vi "Modify Object Owner.vi"(6 "timeout (100 ms)":i32, 10 "UniqueName Object":refnum<class "UniqueName.lvclass">, 11 "New Parent Fully Qualified Name":string) -> (0 "timed out":bool, 1 "operation complete":bool, 2 "Modified UniqueName Object":refnum<class "UniqueName.lvclass">)   [LabVIEW 2014, in "UniqueName.lvlib" / "UniqueName.lvclass"]
uses:
  UniqueName.lvclass
  Command.ctl
  UniquenessCriteria/UniquenessCriteria.lvclass/UniquenessCriteria.ctl
  UniqueName.lvclass/UniqueName.ctl
  Key.ctl
  UniquenessCriteria/UniquenessCriteria.lvclass
  NameIncrementAlgorithm/StringIncrementAlgorithm.lvclass
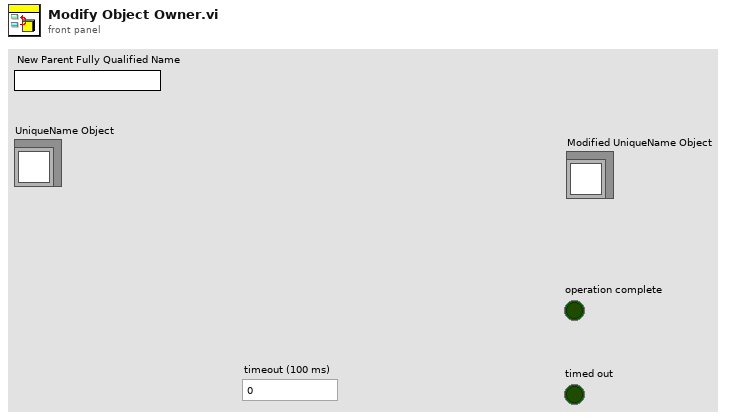
[diagram p1: front panel]
types:
  T1 = typedef "UniqueName.lvlib/UniqueName.lvclass/Command.ctl" = enum16{"Get", "Get All", "Set", "Delete", "Get Status", "Init", "Reserve Ownership", "Release Ownership", "Lock", "Unlock"}
  T2 = typedef "UniqueName.lvlib/UniqueName.lvclass/RegistryStatus.ctl" = cluster{"Registry Configuration":T3, "Registry Owned":bool, "Write-Protected":bool, "Owned":bool, "Released":bool, "Locked":bool, "Unlocked":bool}
  T3 = typedef "UniqueName.lvlib/UniqueName.lvclass/RegistryConfiguration.ctl" = cluster{"Delimiter":refnum<class "Delimiter.lvclass">, "RandomStringGenerator":refnum<class "RandomStringGenerator.lvclass">, "UniquenessCriteria":refnum<class "UniquenessCriteria.lvclass">, "StringIncrement":refnum<class "StringIncrementAlgorithm.lvclass">}
  T4 = typedef "UniqueName.lvlib/UniqueName.lvclass/Key.ctl" = enum16{"Fully Qualified Name", "Unique Name", "Given Name", "Parent Fully Qualified Name"}
  T5 = typedef "UniqueName.lvlib/UniquenessCriteria.lvclass/Criteria.ctl" = enum16{"Globally-Unique Fully Qualified Name", "Globally-Unique Name"}
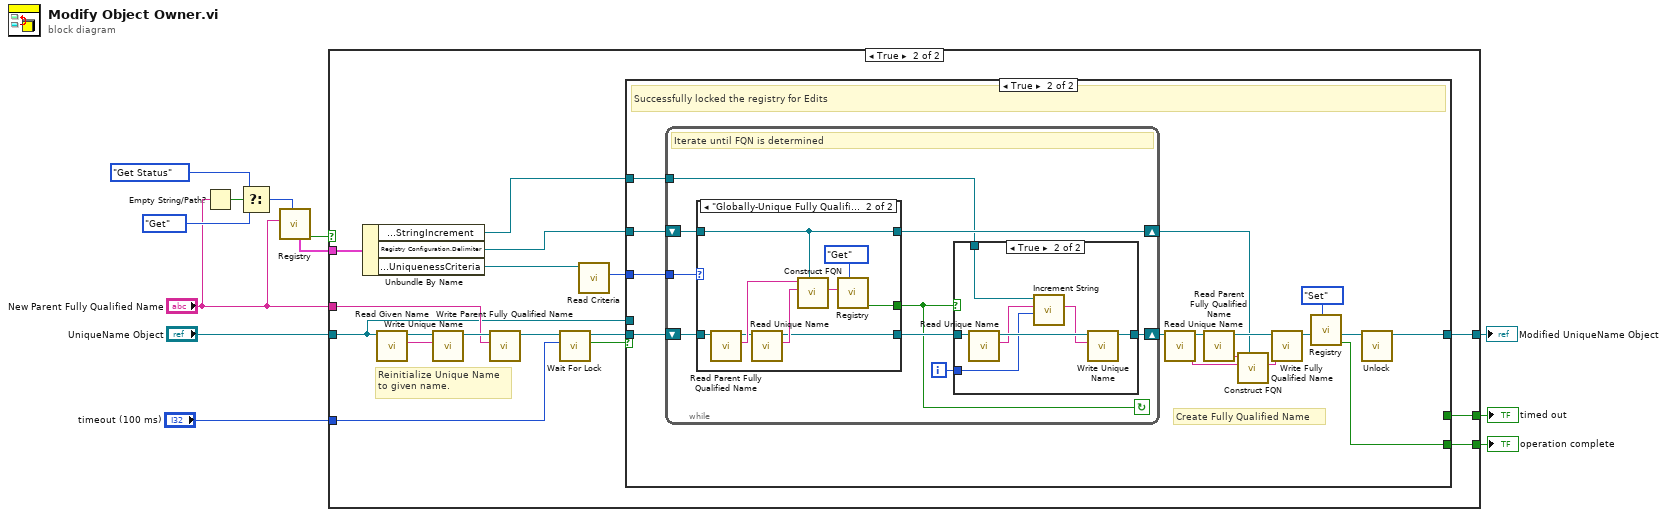
[diagram p0: block diagram]
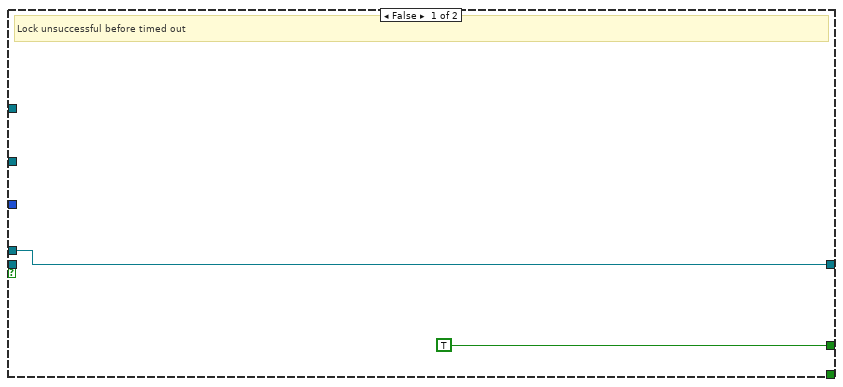
[diagram p3: hidden frame]
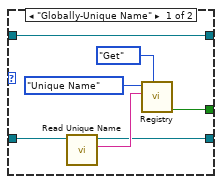
[diagram p5: hidden frame]
diagram:
  n1 = Empty String/Path?(string/path="New Parent Fully Qualified Name") -> (empty?=w8:bool)
  n2 = Select(t=Command."Get Status" ("Command (Get)"), s=w8, f=Command."Get" ("Command (Get)")) -> (s? t:f=w5:T1)
  n3 = call "Registry.vi"("Command (Get)"=w5, "Search term (Get & Delete Operations)"="New Parent Fully Qualified Name") -> ("Found or Completed?"=w3:bool, "Registry Status"=w10:T2)  [unwired: 5 in, 3 out]
  n4 = case shown="True" w3 {
    tunnel: [w13 w29] -> w12
    tunnel: [_ w27] -> w11
    tunnel: w10 -> [_ w26]
    tunnel: "timeout (100 ms)" -> [_ w24]
    tunnel: "UniqueName Object" -> [w13 w14]
    tunnel: "New Parent Fully Qualified Name" -> [_ w18]
    tunnel: [_ w17] -> w2
    frame False {
    }
    frame True {
      # "Reinitialize Unique Name\nto given name."
      n5 = Unbundle By Name(w26) -> ("Registry Configuration.StringIncrement"=w21:refnum<class "StringIncrementAlgorithm.lvclass">, "Registry Configuration.Delimiter"=w22:refnum<class "Delimiter.lvclass">, "Registry Configuration.UniquenessCriteria"=w23:refnum<class "UniquenessCriteria.lvclass">)
      n6 = call "Read Given Name.vi"("UniqueName in"=w14) -> ("Given Name"=w15:string, "UniqueName out"=w16:refnum<class "UniqueName.lvclass">)  [unwired: 9 in]
      n7 = call "Write Unique Name.vi"("Unique Name"=w15, "UniqueName in"=w16) -> ("UniqueName out"=w30:refnum<class "UniqueName.lvclass">)  [unwired: 9 in]
      n8 = call "Write Parent Fully Qualified Name.vi"("Parent Fully Qualified Name"=w18, "UniqueName in"=w30) -> ("UniqueName out"=w19:refnum<class "UniqueName.lvclass">)  [unwired: 9 in]
      n9 = call "Wait For Lock.vi"("timeout (100 ms)"=w24, "UniqueName in"=w19) -> ("Locked"=w28:bool, "UniqueName out"=w20:refnum<class "UniqueName.lvclass">)  [unwired: 8 in]
      n10 = call "Read Criteria.vi"("UniquenessCriteria in"=w23) -> ("Criteria"=w25:T5)  [unwired: 9 in, 1 out]
      n11 = case shown="True" w28 {
        tunnel: w25 -> [_ w47]
        tunnel: w20 -> [_ w40]
        tunnel: [w31 w37] -> w29
        tunnel: [TRUE _] -> w27
        tunnel: w22 -> [_ w36]
        tunnel: w21 -> [_ w35]
        tunnel: [_ w33] -> w17
        tunnel: w14 -> [w31 _]
        frame False {
          # "Lock unsuccessful before timed out"
        }
        frame True {
          # "Create Fully Qualified Name"
          # "Successfully locked the registry for Edits"
          n12 = while {
            tunnel: w47 -> [w57]
            shift-right: [w55] -> w43
            shift-left: w40 -> [w54]
            shift-right: [w51] -> w39
            shift-left: w36 -> [w52]
            tunnel: w35 -> [w50]
            i -> [w49]
            stop <- w53 continue-if-true
            # "Iterate until FQN is determined"
            n13 = case shown="\"Globally-Unique Fully Qualified Name\"" w57 {
              tunnel: [w70 w80] -> w53
              tunnel: w54 -> [w69 w75]
              tunnel: [w67 w73] -> w56
              tunnel: w52 -> [w66 w76]
              tunnel: [w66 w76] -> w51
              frame "Globally-Unique Name" {
                n14 = call "Read Unique Name.vi"("UniqueName in"=w69) -> ("Unique Name"=w68:string, "UniqueName out"=w67:refnum<class "UniqueName.lvclass">)  [unwired: 9 in]
                n15 = call "Registry.vi"("Command (Get)"=Command."Get", "Search term (Get & Delete Operations)"=w68, "Key (FQN)"=Key."Unique Name") -> ("Found or Completed?"=w70:bool)  [unwired: 4 in, 4 out]
              }
              frame "Globally-Unique Fully Qualified Name" {
                n16 = call "Read Parent Fully Qualified Name.vi"("UniqueName in"=w75) -> ("Parent Fully Qualified Name"=w78:string, "UniqueName out"=w74:refnum<class "UniqueName.lvclass">)  [unwired: 9 in]
                n17 = call "Read Unique Name.vi"("UniqueName in"=w74) -> ("Unique Name"=w77:string, "UniqueName out"=w73:refnum<class "UniqueName.lvclass">)  [unwired: 9 in]
                n18 = call "Construct FQN.vi"("Delimiter"=w76, "Name"=w77, "Parent FQN"=w78) -> ("FQN"=w79:string)  [unwired: 8 in]
                n19 = call "Registry.vi"("Command (Get)"=Command."Get", "Search term (Get & Delete Operations)"=w79) -> ("Found or Completed?"=w80:bool)  [unwired: 5 in, 4 out]
              }
            }
            n20 = case shown="True" w53 {
              tunnel: w56 -> [w58 w64]
              tunnel: [w58 w65] -> w55
              tunnel: w50 -> [_ w62]
              tunnel: w49 -> [_ w59]
              frame False {
                # "Name already unique"
              }
              frame True {
                n21 = call "Read Unique Name.vi"("UniqueName in"=w64) -> ("Unique Name"=w61:string, "UniqueName out"=w63:refnum<class "UniqueName.lvclass">)  [unwired: 9 in]
                n22 = call "Increment String.vi"("Numeric"=w59, "Input String"=w61, "String Increment Algorithm"=w62) -> ("Incremented String"=w60:string)  [unwired: 8 in]
                n23 = call "Write Unique Name.vi"("Unique Name"=w60, "UniqueName in"=w63) -> ("UniqueName out"=w65:refnum<class "UniqueName.lvclass">)  [unwired: 9 in]
              }
            }
          }
          n24 = call "Read Unique Name.vi"("UniqueName in"=w43) -> ("Unique Name"=w41:string, "UniqueName out"=w44:refnum<class "UniqueName.lvclass">)  [unwired: 9 in]
          n25 = call "Read Parent Fully Qualified Name.vi"("UniqueName in"=w44) -> ("Parent Fully Qualified Name"=w46:string, "UniqueName out"=w45:refnum<class "UniqueName.lvclass">)  [unwired: 9 in]
          n26 = call "Construct FQN.vi"("Delimiter"=w39, "Name"=w41, "Parent FQN"=w46) -> ("FQN"=w42:string)  [unwired: 8 in]
          n27 = call "Write Fully Qualified Name.vi"("Fully Qualified Name"=w42, "UniqueName in"=w45) -> ("UniqueName out"=w34:refnum<class "UniqueName.lvclass">)  [unwired: 9 in]
          n28 = call "Registry.vi"("Command (Get)"=Command."Set", "UniqueName Object (Set)"=w34) -> ("Found or Completed?"=w33:bool, "Returned Object"=w38:refnum<class "UniqueName.lvclass">)  [unwired: 5 in, 3 out]
          n29 = call "Unlock.vi"("UniqueName in"=w38) -> ("UniqueName out"=w37:refnum<class "UniqueName.lvclass">)  [unwired: 10 in]
        }
      }
    }
  }
  "Modified UniqueName Object" <- w12
  "timed out" <- w11
  "operation complete" <- w2
